vi "wait_opc.vi"(6 "timeout ms (1000)":i32=1000, 8 "error in (no error)":errorcluster, 11 "TCP in":refnum<k5>) -> (0 "error out":errorcluster, 2 "Timeout":bool, 3 "TCP out":refnum<k5>)   [LabVIEW 2025, in "Newtons4thEkg.lvlib"]
uses:
  Newtons4thEkg.lvlib
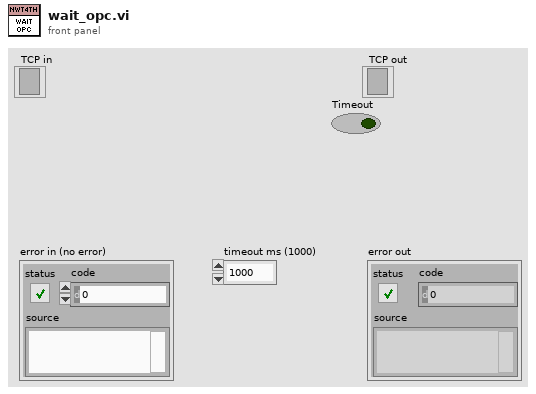
[diagram p1: front panel]
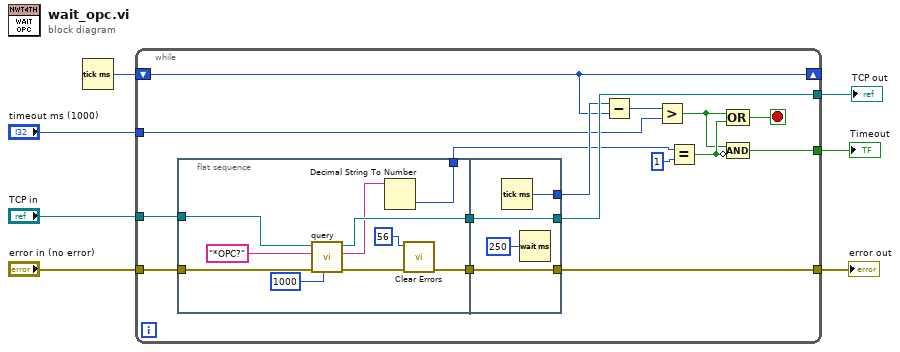
[diagram p0: block diagram]
diagram:
  n1 = Tick Count (ms)() -> (millisecond timer value=w6:u32)
  n2 = while {
    tunnel: "error in (no error)" -> [w23]
    tunnel: [w22] -> w5
    shift-right: [w16] -> _
    shift-left: w6 -> [w16]
    tunnel: "TCP in" -> [w21]
    tunnel: [w20] -> w4
    tunnel: "timeout ms (1000)" -> [w14]
    tunnel: [w9] -> w7
    stop <- w13 stop-if-true
    n3 = flat-sequence {
      tunnel: w23 -> [w33]
      tunnel: w21 -> [w31]
      tunnel: [w25] -> w19
      tunnel: [w30] -> w18
      tunnel: [w26] -> w8
      tunnel: [w36] -> w20
      tunnel: [w37] -> w22
      tunnel: w19 -> [w37]
      tunnel: w18 -> [w36]
      tunnel: [w35] -> w17
      frame #0 {
        n4 = call "query.vi"("timeout ms (1000)"=1000 ("timeout ms (25000)"), "error in (no error)"=w33, "Query"="*OPC?" ("data in"), "TCP in"=w31) -> ("error out"=w32:errorcluster, "Return String"=w28:string, "TCP out"=w30:refnum<k5>)  [unwired: 5 in]
        n5 = Decimal String To Number(string=w28) -> (number=w26:i32)  [unwired: 2 in, 1 out]
        n6 = call <vilib>:"Clear Errors.vi"("error in (no error)"=w32, "specific error code to clear (0: all)"=56) -> ("error out"=w25:errorcluster)  [unwired: 4 in, 1 out]
      }
      frame #1 {
        n7 = Tick Count (ms)() -> (millisecond timer value=w35:u32)
        n8 = Wait (ms)(milliseconds to wait=u32 250) -> ()  [unwired: 1 out]
      }
    }
    n9 = Subtract(x=w17, y=w16) -> (x-y=w15:u32)
    n10 = Greater?(x=w15, y=w14) -> (0:w10:bool)
    n11 = Equal?(x=w8, y=1) -> (x = y?=w11:bool)
    n12 = Compound Arithmetic op=OR(w10, w11) -> (w13:bool)
    n13 = Compound Arithmetic op=AND(w10, invert w11) -> (w9:bool)
  }
  "TCP out" <- w4
  "error out" <- w5
  "Timeout" <- w7
